vi "TYPES OF CONTROLS AND INDICATOR.vi"() -> ()   [LabVIEW 2020]
panel:
  out "Meter":dbl(knob) scale=0.0..10.0
  out "Horizontal Pointer slide Control":dbl(slide) scale=0.0..10.0
  in  "Vertical pointer Slilde Control":dbl(slide) scale=0.0..10.0
  in  "Thermometer":dbl(slide) scale=0.0..100.0
  in  "Tank":dbl(slide) scale=0.0..10.0
  out "Numeric":dbl
  out "Numeric Indicator":dbl
  out "Gauge":dbl(knob) scale=0.0..10.0
  in  "Dial":dbl(knob) scale=0.0..10.0
  out "String Indicator":string
  in  "String Control":string
  out "Boolean Indicator":bool
  in  "Boolean Control":bool
  out "Numeric Indicator":dbl
  in  "Numeric Control":dbl
  # "TYPES OF CONTROLS AND INDICATORS"
  # "1."
  # "6."
  # "2."
  # "3."
  # "4."
  # "5."
  # "7."
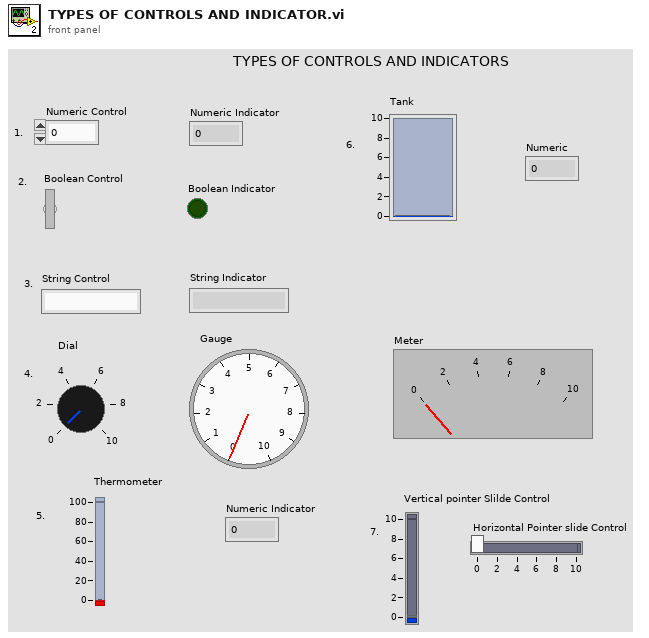
[diagram p1: front panel]
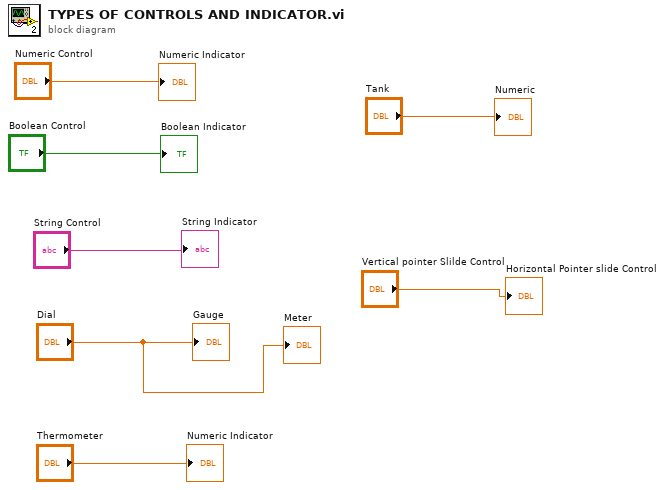
[diagram p0: block diagram]
diagram:
  "Numeric Indicator" <- "Numeric Control"
  "Boolean Indicator" <- "Boolean Control"
  "String Indicator" <- "String Control"
  "Gauge" <- "Dial"
  "Numeric Indicator" <- "Thermometer"
  "Numeric" <- "Tank"
  "Horizontal Pointer slide Control" <- "Vertical pointer Slilde Control"
  "Meter" <- "Dial"
